vi "Parse Multiple Measurements.vi"(10 "Measurement String":string) -> (1 "Measurements Metadata":T1(array[cluster]), 2 "Measurements":dbl[](array[numeric]))   [LabVIEW 2019, in "Keithley 2182.lvlib"]
doc: "Extracts measurement information from string.\n\nReturns two arrays:\n1. Pure numerical values (measurement reading).\n1. Clusters containing metadata for their corresponding numerical value.\n\nSize of both arrays will always be equal.\n\nAssumes all metadata is included in string, which includes:\n\n1. Reading\n2. Unit\n3. Channel\n\n[Mantissa][Exponent][Units], [Channel][Channel Units]\n\ne.g.\n-1.23456789E00VDC, 01INTCHAN"
uses:
  Keithley 2182.lvlib
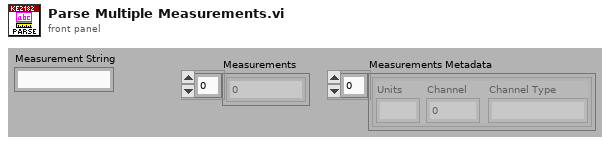
[diagram p1: front panel]
types:
  T1 = cluster{"Units":string, "Channel":i32, "Channel Type":string}[]
  T2 = cluster{"Units":string, "Channel":i32, "Channel Type":string}
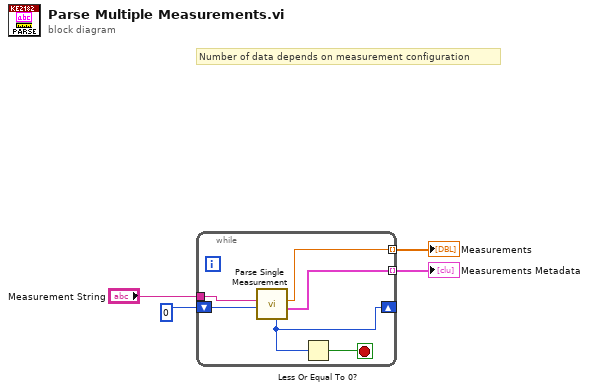
[diagram p0: block diagram]
diagram:
  # "Number of data depends on measurement configuration"
  n1 = while {
    shift-right: [w7] -> _
    shift-left: 0 -> [w9]
    tunnel: "Measurement String" -> [w8]
    tunnel: [w6] -> w2 mode=indexing
    tunnel: [w5] -> w1 mode=indexing
    stop <- w10 stop-if-true
    n2 = call "Parse Single Measurement.vi"("Offset"=w9, "Measurement String"=w8) -> ("Measurement Metadata"=w5:T2, "Measurement"=w6:dbl, "Offset Past Token"=w7:i32)  [unwired: 7 in]
    n3 = Less Or Equal To 0?(x=w7) -> (x <= 0?=w10:bool)
  }
  "Measurements" <- w2
  "Measurements Metadata" <- w1
